vi "Start XNET Sessions.vi"(8 "error in (no error)":errorcluster, 11 "Protocol.Data":T1[](array[typedef]) {"Outgoing.Frames.CountersAndProtections"."Protection Configurations"."CRC Channels"."Data Type" items=["Signed", "Unsigned", "IEEE Float"]; "Trigger.Refs"."Data Reference" format="%.0x"; "Disable.Refs"."Data Reference" format="%.0x"; "Timing.Refs"."Data Reference" format="%.0x"; "Network"."Name" format="%.0x"; "Incoming.Refs"."Data Reference" format="%.0x"; "Outgoing.Refs"."Data Reference" format="%.0x"}) -> (0 "error out":errorcluster, 3 "XNET Sessions":cluster{refnum<k21>[], "Address":u8}[](array[cluster]))   [LabVIEW 2021, in "J1939-22_Engine.lvclass"]
uses:
  J1939-22_Engine.lvclass
  J1939 Addon/Addon/Addon Engine/Types/Protocol.XNET Refs.ctl
  J1939 Addon/Addon/Addon Shared/Types/Monitor Settings.ctl
  <vilib>/NI VeriStand/Custom Device API/Block Data Reference.ctl
  <vilib>/NI VeriStand/Custom Device API/Data Reference.ctl
  J1939 Addon/Addon/Addon Engine/Types/Main.Outgoing.Frame.Settings.ctl
  J1939 Addon/Addon/Addon Shared/Types/Outgoing Event Trigger Types.ctl
  J1939 Addon/SubModules/Frame-Protection-Support/Source/Shared/Types/Exported Frame Settings.ctl
  J1939 Addon/SubModules/Frame-Protection-Support/Source/Shared/Types/Exported Frame Type.ctl
  J1939 Addon/SubModules/Frame-Protection-Support/Source/Shared/Types/Exported Protection Settings.ctl
  J1939 Addon/SubModules/Frame-Protection-Support/Source/Shared/Types/Protection Type.ctl
  J1939 Addon/SubModules/Frame-Protection-Support/Source/Shared/Types/XNET Signal Configuration.ctl
  J1939 Addon/SubModules/Frame-Protection-Support/Source/Shared/Types/Exported Counter Settings.ctl
  J1939 Addon/SubModules/Frame-Protection-Support/Source/Shared/Types/Exported Event Trigger Type.ctl
  <vilib>/xnet/xnet.llb/XNET Control Scope.ctl
  <resource>/objmgr/xnet.rc
  <vilib>/NI VeriStand/Custom Device API/Custom Device API.lvlib
  J1939 Addon/Addon/Addon Shared/J1939 Addon Shared.lvlib
  J1939 Addon/Addon/Addon Engine/J1939 Addon Engine.lvlib
  J1939 Addon/SubModules/Frame-Protection-Support/Source/Shared/Protection and Counter Support Shared.lvlib
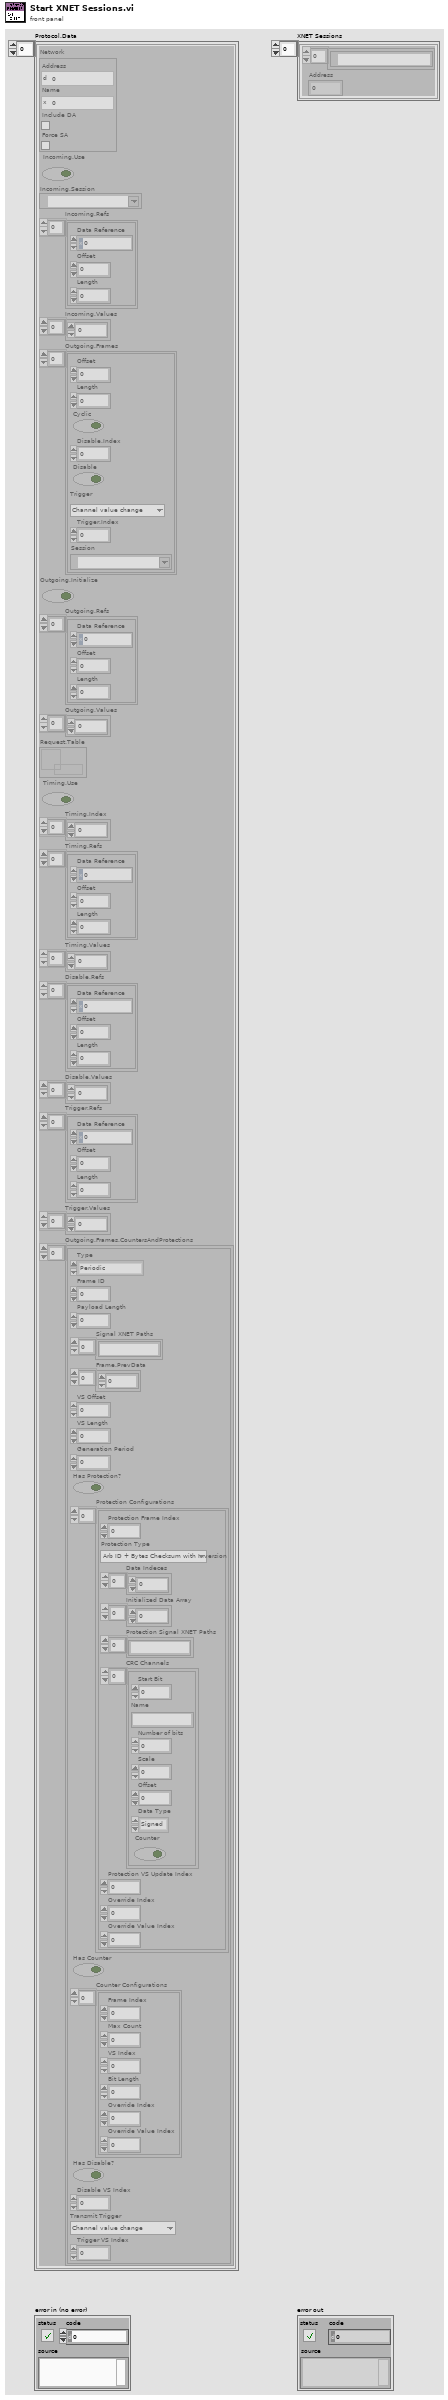
[diagram p1: front panel]
types:
  T1 = typedef "J1939 Addon Engine.lvlib/Protocol.XNET Refs.ctl" = cluster{"Network":T2, "Incoming.Use":bool, "Incoming.Session":refnum<k21>, "Incoming.Refs":T3[], "Incoming.Values":dbl[], "Outgoing.Frames":T5[], "Outgoing.Initialize":bool, "Outgoing.Refs":T3[], "Outgoing.Values":dbl[], "Request.Table":refnum<k33>, "Timing.Use":bool, "Timing.Index":i32[], "Timing.Refs":T3[], "Timing.Values":dbl[], "Disable.Refs":T3[], "Disable.Values":dbl[], "Trigger.Refs":T3[], "Trigger.Values":dbl[], "Outgoing.Frames.CountersAndProtections":T7[]}
  T2 = typedef "J1939 Addon Shared.lvlib/Monitor Settings.ctl" = cluster{"Address":u8, "Name":u64, "Include DA":bool, "Force SA":bool}
  T3 = typedef "Custom Device API.lvlib/Block Data Reference.ctl" = cluster{"Data Reference":T4, "Offset":u64, "Length":u64}
  T4 = typedef "Custom Device API.lvlib/Data Reference.ctl" = i32
  T5 = typedef "J1939 Addon Engine.lvlib/Main.Outgoing.Frame.Settings.ctl" = cluster{"Offset":u32, "Length":u32, "Cyclic":bool, "Disable.Index":i32, "Disable":bool, "Trigger":T6, "Trigger.Index":i32, "Session":refnum<k21>}
  T6 = typedef "J1939 Addon Shared.lvlib/Outgoing Event Trigger Types.ctl" = enum16{"Channel value change", "Trigger channel (not zero)", "Channel value change or trigger channel (not zero)", "Trigger channel (any value change)", "Channel value change or trigger channel (any value change)"}
  T7 = typedef "Protection and Counter Support Shared.lvlib/Exported Frame Settings.ctl" = cluster{"Type":T8, "Frame ID":u32, "Payload Length":u32, "Signal XNET Paths":string[], "Frame.PrevData":dbl[], "VS Offset":i32, "VS Length":i32, "Generation Period":u32, "Has Protection?":bool, "Protection Configurations":T9[], "Has Counter":bool, "Counter Configurations":T12[], "Has Disable?":bool, "Disable VS Index":i32, "Transmit Trigger":T13, "Trigger VS Index":i32}
  T8 = typedef "Protection and Counter Support Shared.lvlib/Exported Frame Type.ctl" = enum16{"Periodic", "Event", "Periodic/Event"}
  T9 = typedef "Protection and Counter Support Shared.lvlib/Exported Protection Settings.ctl" = cluster{"Protection Frame Index":i32, "Protection Type":T10, "Data Indeces":i32[], "Initialized Data Array":dbl[], "Protection Signal XNET Paths":string[], "CRC Channels":T11[], "Protection VS Update Index":i32, "Override Index":i32, "Override Value Index":i32}
  T10 = typedef "Protection and Counter Support Shared.lvlib/Protection Type.ctl" = enum16{"Arb ID + Bytes Checksum with Inversion", "Arb ID + Bytes CRC with Inversion", "Reversed Raw Signal Checksum with Inversion", "Concatenated Two's Compliment"}
  T11 = typedef "Protection and Counter Support Shared.lvlib/XNET Signal Configuration.ctl" = cluster{"Start Bit":i32, "Name":string, "Number of bits":i32, "Scale":dbl, "Offset":dbl, "Data Type":u32, "Counter":bool}
  T12 = typedef "Protection and Counter Support Shared.lvlib/Exported Counter Settings.ctl" = cluster{"Frame Index":i32, "Max Count":dbl, "VS Index":i32, "Bit Length":i64, "Override Index":i32, "Override Value Index":i32}
  T13 = typedef "Protection and Counter Support Shared.lvlib/Exported Event Trigger Type.ctl" = enum16{"Channel value change", "Trigger channel (not zero)", "Channel value change or trigger channel (not zero)", "Trigger channel (any value change)", "Channel value change or trigger channel (any value change)"}
  T14 = typedef "XNET Control Scope.ctl" = u32
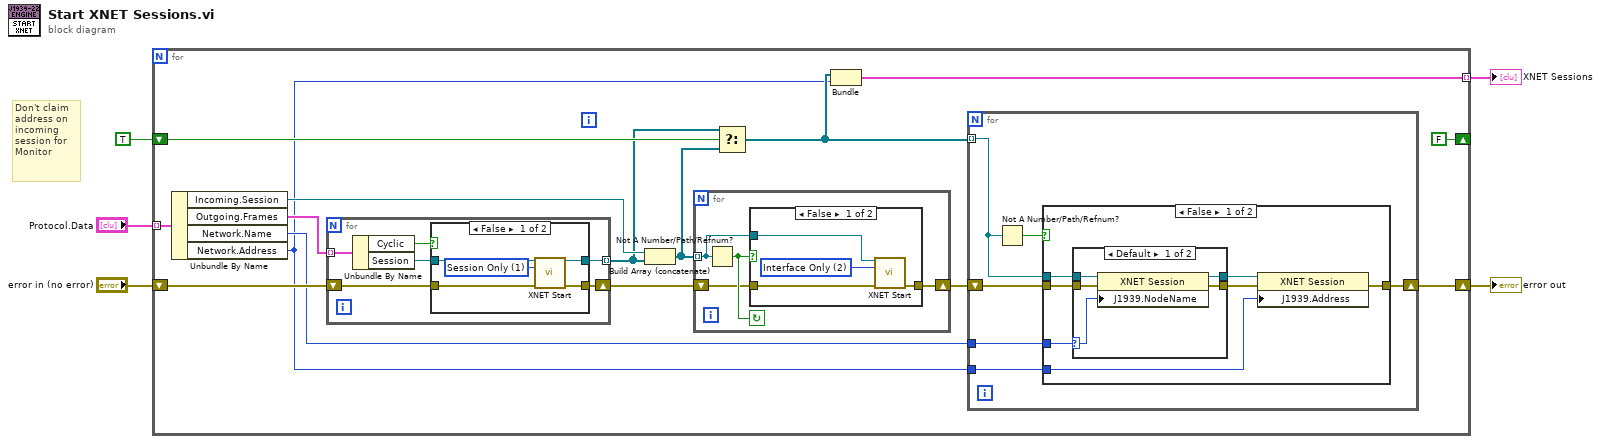
[diagram p0: block diagram]
diagram:
  # "Don't claim address on incoming session for Monitor"
  n1 = for {
    shift-right: [w14] -> w4
    shift-left: "error in (no error)" -> [w19]
    tunnel: "Protocol.Data" -> [w18] mode=indexing
    shift-right: [FALSE] -> _
    shift-left: TRUE -> [w12]
    tunnel: [w6] -> w5 mode=indexing
    n2 = Unbundle By Name(w18) -> ("Incoming.Session"=w17:refnum<k21>, "Outgoing.Frames"=w20:T5[], "Network.Name"=w13:u64, "Network.Address"=w7:u8)
    n3 = for {
      tunnel: w20 -> [w35] mode=indexing
      shift-right: [w33] -> w16
      shift-left: w19 -> [w34]
      tunnel: [w32] -> w11 mode=indexing
      n4 = Unbundle By Name(w35) -> ("Cyclic"=w30:bool, "Session"=w31:refnum<k21>)
      n5 = case shown="False" w30 {
        tunnel: w34 -> [w40 w41]
        tunnel: [w39 w41] -> w33
        tunnel: [w38 w42] -> w32
        tunnel: w31 -> [w37 w42]
        frame False {
          w36 = T14 1 items=["Normal", "Session Only", "Interface Only", "Session Only Blocking"] ("scope (normal)")
          n6 = call <vilib>:"XNET Start.vi"("session in"=w37, "scope (normal)"=w36, "error in (no error)"=w40) -> ("session out"=w38:refnum<k21>, "error out"=w39:errorcluster)  [unwired: 11 in]
        }
        frame True {
        }
      }
    }
    n7 = Build Array (concatenate)(w17, w11) -> (w10:refnum<k21>[])
    n8 = for {
      tunnel: w10 -> [w22] mode=indexing
      shift-right: [w21] -> w15
      shift-left: w16 -> [w23]
      stop <- w24 continue-if-true
      n9 = Not A Number/Path/Refnum?(number/path/refnum=w22) -> (NaN/Path/Refnum?=w24:bool)
      n10 = case shown="False" w24 {
        tunnel: w23 -> [w26 w29]
        tunnel: w22 -> [w27 _]
        tunnel: [w25 w29] -> w21
        frame False {
          w28 = T14 2 items=["Normal", "Session Only", "Interface Only", "Session Only Blocking"] ("scope (normal)")
          n11 = call <vilib>:"XNET Start.vi"("session in"=w27, "scope (normal)"=w28, "error in (no error)"=w26) -> ("error out"=w25:errorcluster)  [unwired: 11 in, 1 out]
        }
        frame True {
        }
      }
    }
    n12 = Select(t=w11, s=w12, f=w10) -> (s? t:f=w8:refnum<k21>[])
    n13 = Bundle(w8, "Address"=w7) -> (w6:cluster{refnum<k21>[], "Address":u8})  [unwired: 1 in]
    n14 = for {
      tunnel: w8 -> [w46] mode=indexing
      shift-right: [w45] -> w14
      shift-left: w15 -> [w47]
      tunnel: w13 -> [w44]
      tunnel: w7 -> [w43]
      n15 = Not A Number/Path/Refnum?(number/path/refnum=w46) -> (NaN/Path/Refnum?=w48:bool)
      n16 = case shown="False" w48 {
        tunnel: w47 -> [w54 w63]
        tunnel: w46 -> [w55 _]
        tunnel: [w53 w63] -> w45
        tunnel: w44 -> [w50 _]
        tunnel: w43 -> [w51 _]
        frame False {
          n17 = case shown="Default" w50 {
            selector: w50 -> [w58 _]
            tunnel: w55 -> [w60 w61]
            tunnel: w54 -> [w59 w62]
            tunnel: [w57 w62] -> w52
            tunnel: [w56 w61] -> w49
            frame Default {
              n18 = property class="XNET Session"(reference=w60, error in=w59, "J1939.NodeName"=w58) -> (reference out=w56:refnum<k21>, error out=w57:errorcluster)
            }
            frame 0 {
            }
          }
          n19 = property class="XNET Session"(reference=w49, error in=w52, "J1939.Address"=w51) -> (error out=w53:errorcluster)  [unwired: 1 out]
        }
        frame True {
        }
      }
    }
  }
  "XNET Sessions" <- w5
  "error out" <- w4
